vi "Panel Resized.vi"(6 "Sizing Refnums":T2, 8 "error in (no error)":errorcluster, 9 "Origin":cluster{"H":i16, "V":i16}, 10 "NewBnds":T1, 11 "Size Constraints":cluster{"min tab width":i32, "w/h":dbl}) -> (0 "error out":errorcluster)   [LabVIEW 2014]
uses:
  <vilib>/Utility/miscctls.llb/LVRectTypeDef.ctl
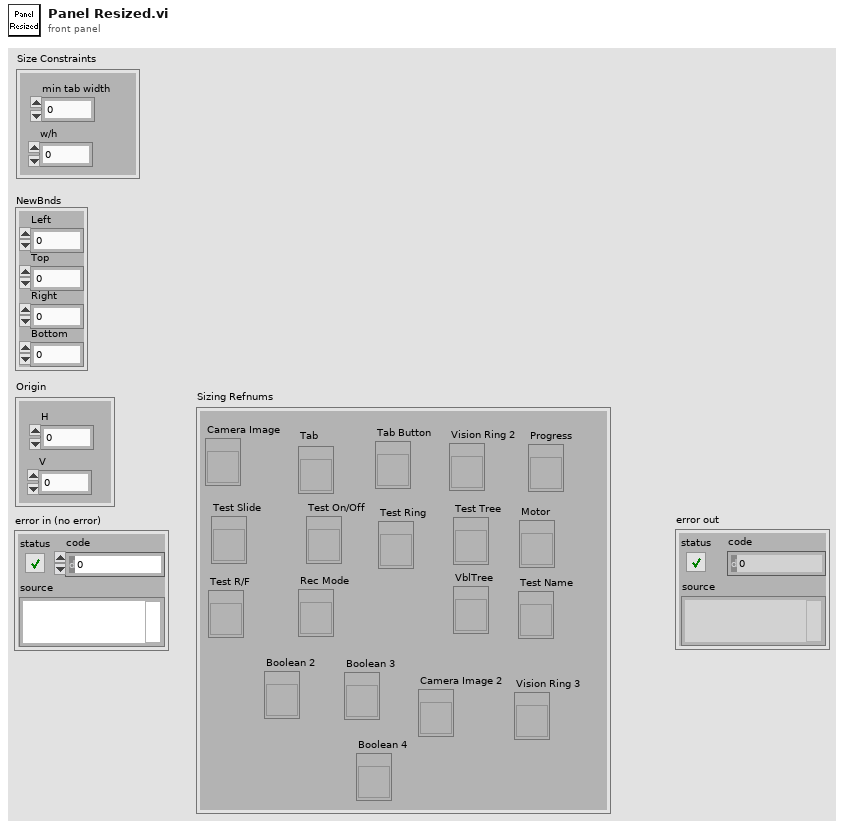
[diagram p1: front panel]
types:
  T1 = typedef "LVRectTypeDef.ctl" = cluster{"Left":i16, "Top":i16, "Right":i16, "Bottom":i16}
  T2 = cluster{"Camera Image":refnum<vi>, "Tab":refnum<vi>, "Tab Button":refnum<vi>, "Vision Ring 2":refnum<vi>, "Rec Mode":refnum<vi>, "Test Slide":refnum<vi>, "Test On/Off":refnum<vi>, "Test Ring":refnum<vi>, "Test R/F":refnum<vi>, "Test Name":refnum<vi>, "Motor":refnum<vi>, "Progress":refnum<vi>, "Test Tree":refnum<vi>, "VblTree":refnum<vi>, "Boolean 2":refnum<vi>, "Boolean 3":refnum<vi>, "Camera Image 2":refnum<vi>, "Vision Ring 3":refnum<vi>, "Boolean 4":refnum<vi>}
  T3 = typedef "LVPositionTypeDef.ctl" = cluster{"Left":i32, "Top":i32}
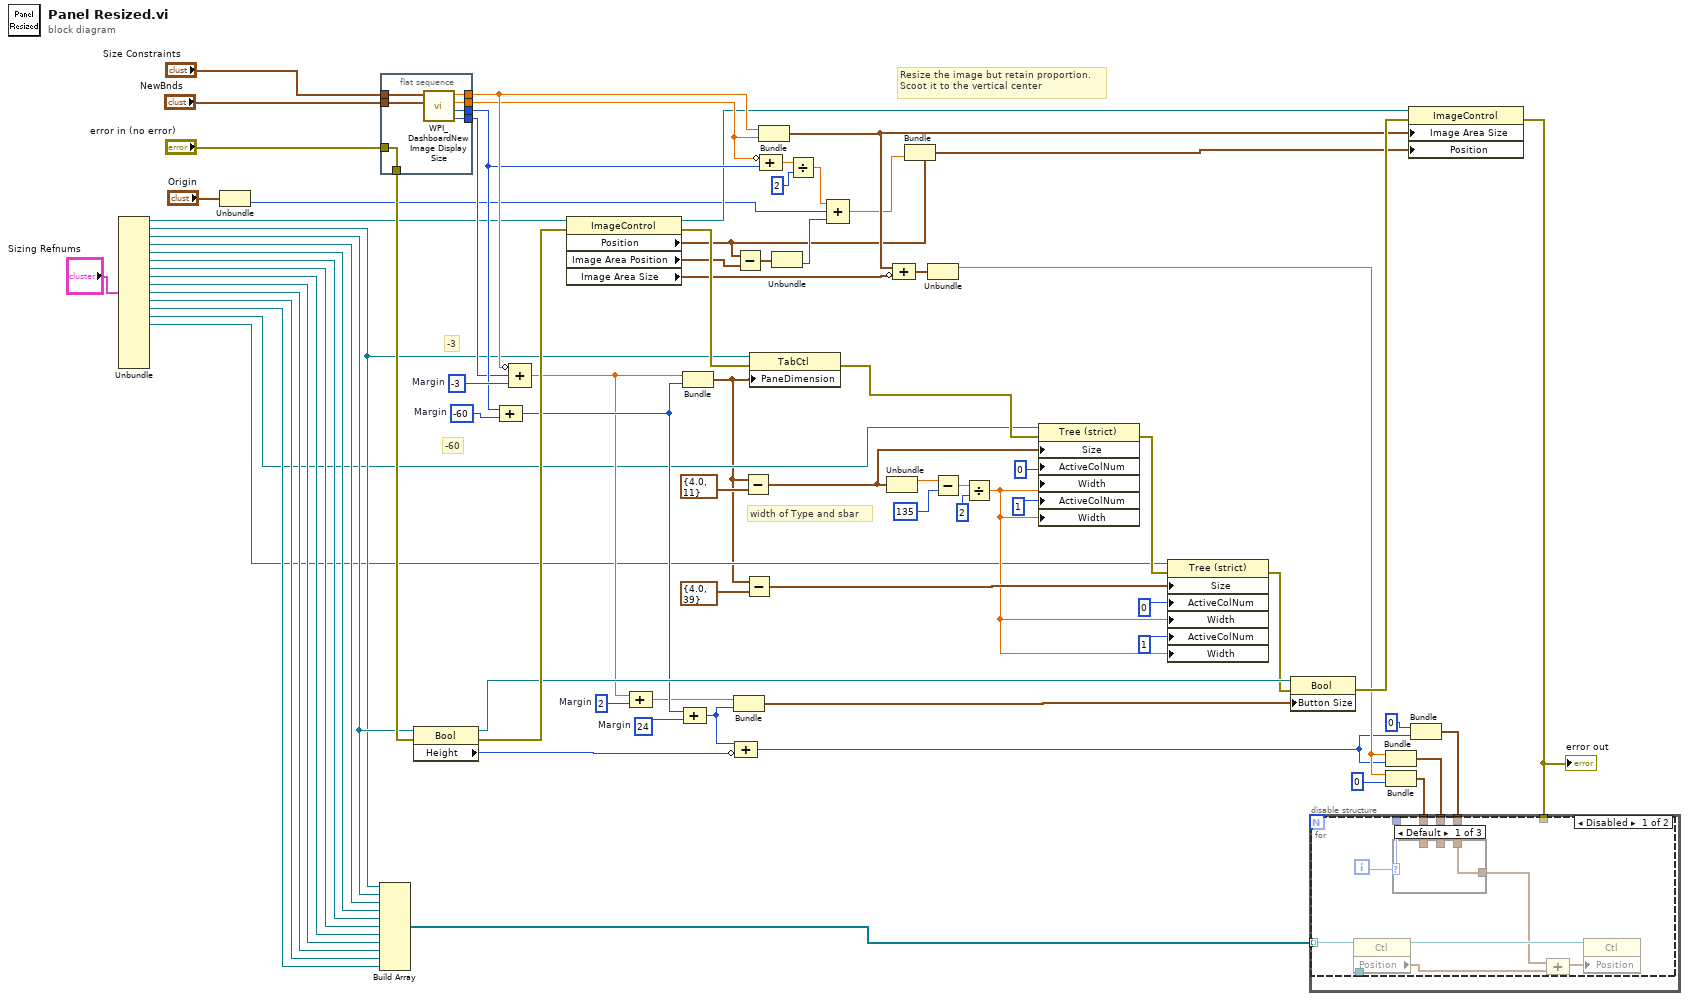
[diagram p0: block diagram]
diagram:
  w58 = 24  # Margin
  w56 = 2  # Margin
  w52 = -60  # Margin
  w62 = -3  # Margin
  # "-60"
  # "-3"
  # "width of Type and sbar"
  # "Resize the image but retain proportion.\nScoot it to the vertical center"
  n1 = Unbundle("Sizing Refnums") -> ("Camera Image"=w27:refnum<vi>, "Tab"=w28:refnum<vi>, "Tab Button"=w35:refnum<vi>, "Vision Ring 2"=w73:refnum<vi>, "Rec Mode"=w74:refnum<vi>, "Test Slide"=w75:refnum<vi>, "Test On/Off"=w76:refnum<vi>, "Test Ring"=w77:refnum<vi>, "Test R/F"=w78:refnum<vi>, "Test Name"=w11:refnum<vi>, "Motor"=w10:refnum<vi>, "Progress"=w6:refnum<vi>, "Test Tree"=w4:refnum<vi>, "VblTree"=w3:refnum<vi>)  [unwired: 5 out]
  n2 = Unbundle("Origin") -> ("V"=w33:i16)  [unwired: 1 out]
  n3 = Build Array(w28, w35, w73, w74, w75, w76, w77, w78, w11, w10, w6) -> (w72:refnum<vi>[])
  n4 = flat-sequence {
    tunnel: "NewBnds" -> [w85]
    tunnel: "Size Constraints" -> [w84]
    tunnel: [w83] -> w51
    tunnel: [w82] -> w59
    tunnel: [w81] -> w60
    tunnel: [w80] -> w61
    tunnel: [w79] -> w71
    tunnel: "error in (no error)" -> [w79]
    frame #0 {
      n5 = call <vilib>:"WPI_DashboardNew Image Display Size.vi"("NewBnds"=w85, "Size Constraints"=w84) -> ("Window Width"=w83:i16, "Window Height"=w81:i16, "Height"=w82:dbl, "Width"=w80:dbl)  [unwired: 6 in]
    }
  }
  n6 = property class="Bool"(reference=w35, error in=w71) -> (reference out=w65:refnum<vi>, error out=w70:errorcluster, "Height"=w64:u32)
  n7 = Compound Arithmetic op=unknown(w60, w52) -> (w57:i32)
  n8 = Compound Arithmetic op=ADD(invert w61, w51, w62) -> (w55:dbl)
  n9 = property class="ImageControl"(reference=w27, error in=w70) -> (reference out=w44:refnum<vi>, error out=w68:errorcluster, "Position"=w43:T3, "Image Area Position"=w38:cluster{"Left":i32, "Top":i32}, "Image Area Size"=w49:cluster{"Width":u32, "Height":u32})
  n10 = Compound Arithmetic op=ADD(w55, w56) -> (w54:dbl)
  n11 = Bundle(w55, w57) -> (w2:cluster{dbl, i32})  [unwired: 1 in]
  n12 = Compound Arithmetic op=ADD(w57, w58) -> (w63:i32)
  n13 = Bundle(w54, w63) -> (w53:cluster{dbl, i32})  [unwired: 1 in]
  n14 = Subtract(x=w43, y=w38) -> (x-y=w45:T3)
  n15 = Compound Arithmetic op=ADD(w63, invert w64) -> (w9:u32)
  n16 = Subtract(x=w2, y=cluster{dbl, i32} {4.0, 11}) -> (x-y=w19:cluster{dbl, i32})
  n17 = Subtract(x=w2, y=cluster{dbl, i32} {4.0, 39}) -> (x-y=w24:cluster{dbl, i32})
  n18 = property class="TabCtl"(reference=w28, error in=w68, "PaneDimension"=w2) -> (error out=w5:errorcluster)  [unwired: 1 out]
  n19 = Bundle("Width"=w61, "Height"=w59) -> (w47:cluster{"Width":dbl, "Height":dbl})  [unwired: 1 in]
  n20 = Compound Arithmetic op=ADD(invert w59, w60) -> (w39:dbl)
  n21 = Unbundle(w45) -> ("Top"=w46:i32)  [unwired: 1 out]
  n22 = Divide(x=w39, y=2) -> (x/y=w41:dbl)
  n23 = Compound Arithmetic op=ADD(w41, w33, w46) -> (w42:dbl)
  n24 = Unbundle(w19) -> (w18:dbl)  [unwired: 1 out]
  n25 = Compound Arithmetic op=ADD(w47, invert w49) -> (w50:cluster{"Width":dbl, "Height":dbl})
  n26 = Bundle(cluster=w43, "Top"=w42) -> (w48:T3)  [unwired: 1 in]
  n27 = Unbundle(w50) -> ("Width"=w66:dbl)  [unwired: 1 out]
  n28 = Subtract(x=w18, y=135 ("Active Cell:Active Column Number")) -> (x-y=w14:dbl)
  n29 = Divide(x=w14, y=2 ("Active Cell:Active Column Number")) -> (x/y=w12:dbl)
  n30 = property class="Tree (strict)"(reference=w4, error in=w5, "Size"=w19, "ActiveColNum"=0 ("Active Cell:Active Column Number"), "Width"=w12, "ActiveColNum"=1 ("Active Cell:Active Column Number"), "Width"=w12) -> (error out=w23:errorcluster)  [unwired: 1 out]
  n31 = property class="Tree (strict)"(reference=w3, error in=w23, "Size"=w24, "ActiveColNum"=0 ("Active Cell:Active Column Number"), "Width"=w12, "ActiveColNum"=1 ("Active Cell:Active Column Number"), "Width"=w12) -> (error out=w22:errorcluster)  [unwired: 1 out]
  n32 = property class="Bool"(reference=w65, error in=w22, "Button Size"=w53) -> (error out=w69:errorcluster)  [unwired: 1 out]
  n33 = Bundle("Width"=w66, w9) -> (w37:cluster{"Width":dbl, u32})  [unwired: 1 in]
  n34 = Bundle("Width"=w66, 0) -> (w36:cluster{"Width":dbl, i32})  [unwired: 1 in]
  n35 = property class="ImageControl"(reference=w44, error in=w69, "Image Area Size"=w47, "Position"=w48) -> (error out=w32:errorcluster)  [unwired: 1 out]
  "error out" <- w32
  n36 = Bundle(0, w9) -> (w7:cluster{i32, u32})  [unwired: 1 in]
  n37 = for {
    tunnel: w72 -> [w90] mode=indexing
    tunnel: w37 -> [w87]
    tunnel: w36 -> [w88]
    tunnel: w32 -> [_]
    tunnel: w7 -> [w86]
    i -> [w89]
    n38 = disable-structure shown="Disabled" {
      disable-tunnel: w90 -> [w99 _]
      disable-tunnel: w89 -> [w95 _]
      disable-tunnel: w88 -> [w94 _]
      disable-tunnel: w87 -> [w93 _]
      disable-tunnel: w86 -> [w92 _]
      frame Disabled {
        n39 = property class="Ctl"(reference=w99) -> (reference out=w98:refnum<vi>, "Position"=w97:T3)  [unwired: 1 in, 1 out]
        n40 = case shown="Default" w95 {
          tunnel: w94 -> [_ w101 _]
          tunnel: w93 -> [_ _ w102]
          tunnel: w92 -> [w100 _ _]
          tunnel: [w100 w101 w102] -> w91
          frame Default {
          }
          frame 0, 1 {
          }
          frame 2, 3 {
          }
        }
        n41 = Compound Arithmetic op=ADD(w91, w97) -> (w96:cluster{dbl, u32})
        n42 = property class="Ctl"(reference=w98, "Position"=w96) -> ()  [unwired: 1 in, 2 out]
      }
      frame Enabled {
      }
    }
  }
